vi "5668 Get Array Index from Frequency Value.vi"(9 "df":dbl, 10 "f0":dbl, 11 "Numeric Control in":dbl) -> (3 "Numeric Control out":i32)   [LabVIEW 2017]
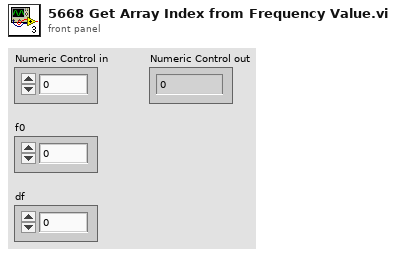
[diagram p1: front panel]
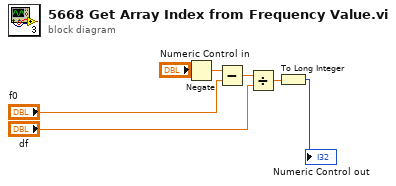
[diagram p0: block diagram]
diagram:
  n1 = Negate(x="Numeric Control in") -> (-x=w6:dbl)
  n2 = Subtract(x=w6, y="f0") -> (x-y=w5:dbl)
  n3 = Divide(x=w5, y="df") -> (x/y=w4:dbl)
  n4 = To Long Integer(number=w4) -> (32bit integer=→"Numeric Control out":i32)
